vi "array_concatenate.vi"() -> ()   [LabVIEW 2012]
panel:
  out "波形图表":i32[](graph)
  out "波形图":i32[][](graph)
  out "数组":i32[][](array[numeric])
  out "数值":dbl
  out "数组 2":dbl[](array[numeric])
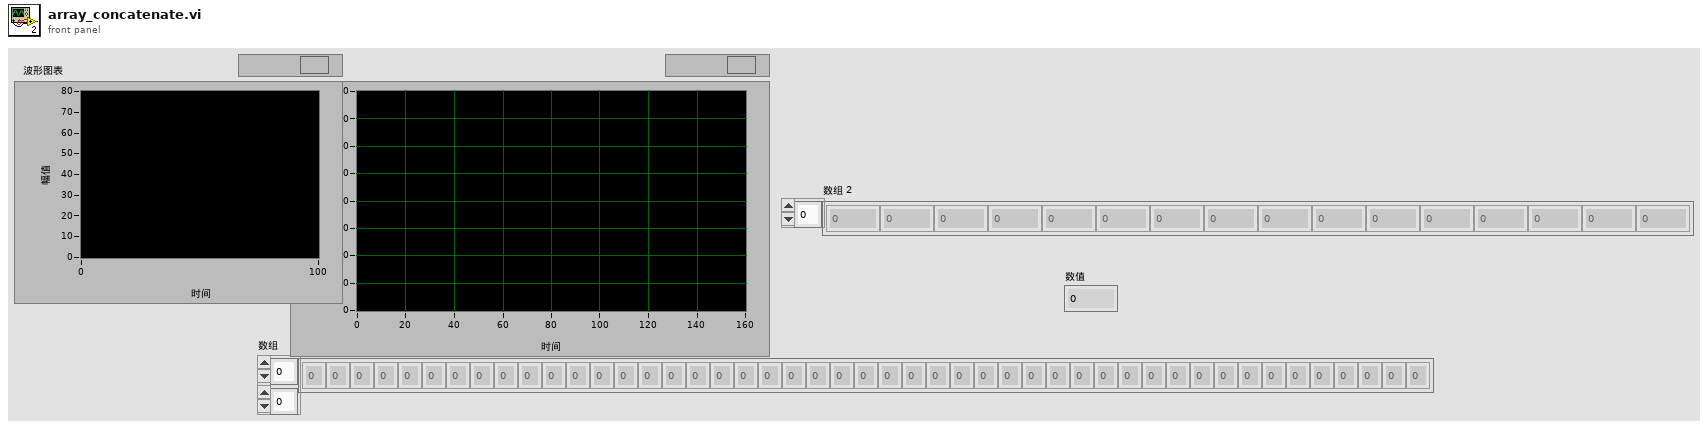
[diagram p1: front panel]
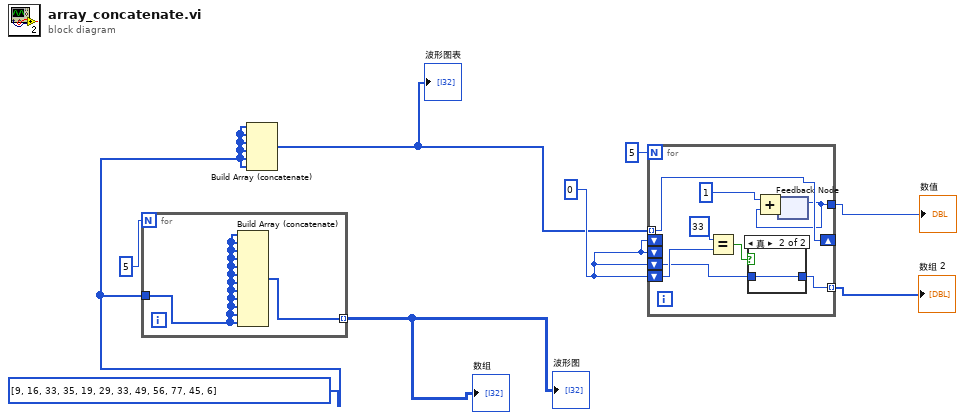
[diagram p0: block diagram]
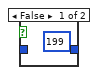
[diagram p2: hidden frame]
diagram:
  w2 = i32[] [9, 16, 33, 35, 19, 29, 33, 49, 56, 77, 45, 6] ("数组 3")
  w8 = 0
  n1 = for {
    N: 5 -> [_]
    tunnel: w2 -> [w9]
    tunnel: [w10] -> w3 mode=indexing
    n2 = Build Array (concatenate)(w9, w9, w9, w9, w9, w9, w9, w9, w9, w9, w9, w9) -> (w10:i32[])
  }
  "数组" <- w3
  "波形图" <- w3
  n3 = Build Array (concatenate)(w2, w2, w2, w2, w2, w2) -> (w1:i32[])
  "波形图表" <- w1
  n4 = for {
    N: 5 -> [_]
    shift-right: [w17] -> _
    shift-left: w8 -> [_]
    shift-left: w8 -> [_]
    shift-left: w8 -> [w14]
    shift-left: w8 -> [w16]
    tunnel: w1 -> [w17] mode=indexing
    tunnel: [w15] -> w7 mode=indexing
    tunnel: [w11] -> w6
    n5 = Equal?(x=33, y=w16) -> (x = y?=w18:bool)
    n6 = case shown="真" w18 {
      tunnel: w14 -> [_ w21]
      tunnel: [199 w21] -> w15
      frame False {
      }
      frame True {
      }
    }
    n7 = feedback #1() -> (w11:i32)  [unwired: 1 in]
    n8 = Add(x=1, y=w11) -> (x+y=w12:i32)
    n9 = feedback-in #1(w12) -> ()
  }
  "数组 2" <- w7
  "数值" <- w6
